vi "DSF.Engine.Hardware Info.CPU.Get Core Count.vi"(8 "error in (no error)":errorcluster, 11 "CPU Info in":refnum<class "DSF.Engine.Hardware Info.CPU.lvclass">) -> (0 "error out":errorcluster, 2 "Core Count":i32, 3 "CPU Info out":refnum<class "DSF.Engine.Hardware Info.CPU.lvclass">)   [LabVIEW 2017, in "DSF.Engine.lvlib" / "DSF.Engine.Hardware Info.CPU.lvclass"]
uses:
  DSF.Engine.Hardware Info.CPU.lvclass
  DSF.Engine.Hardware Info.CPU.lvclass/DSF.Engine.Hardware Info.CPU.ctl
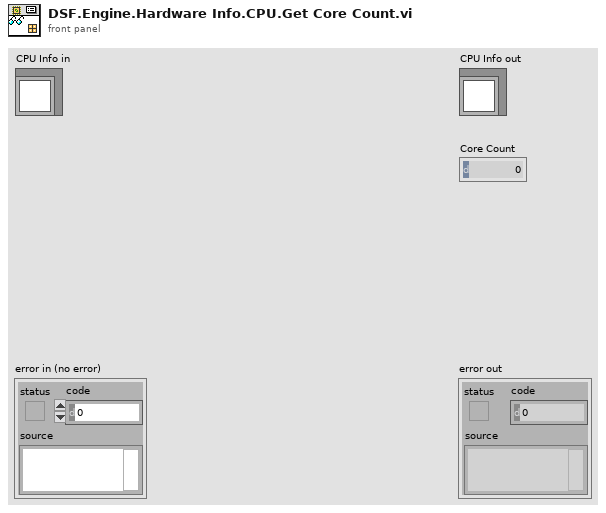
[diagram p1: front panel]
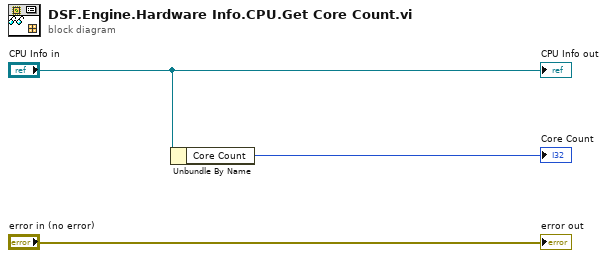
[diagram p0: block diagram]
diagram:
  n1 = Unbundle By Name("CPU Info in") -> ("Core Count"=→"Core Count":i32)
  "error out" <- "error in (no error)"
  "CPU Info out" <- "CPU Info in"
